vi "Main.Write Data to VS.vi"(8 "error in":errorcluster, 11 "Data Sessions":T1[](array[typedef]) {"Trigger.Refs"."Data Reference" format="%.0x"; "Disable.Refs"."Data Reference" format="%.0x"; "Timing.Refs"."Data Reference" format="%.0x"; "Network"."Name" format="%.0x"; "Incoming.Refs"."Data Reference" format="%.0x"; "Outgoing.Refs"."Data Reference" format="%.0x"}) -> (0 "error out":errorcluster, 3 "Data Sessions out":T1[](array[typedef]) {"Trigger.Refs"."Data Reference" format="%.0x"; "Disable.Refs"."Data Reference" format="%.0x"; "Timing.Refs"."Data Reference" format="%.0x"; "Network"."Name" format="%.0x"; "Incoming.Refs"."Data Reference" format="%.0x"; "Outgoing.Refs"."Data Reference" format="%.0x"})   [LabVIEW 2015, in "J1939 Addon Engine.lvlib"]
uses:
  J1939 Addon Engine.lvlib
  Types/Protocol.XNET Refs.ctl
  Shared/Types/Monitor Settings.ctl
  <vilib>/NI Veristand/Custom Device API/Block Data Reference.ctl
  <vilib>/NI Veristand/Custom Device API/Data Reference.ctl
  Types/Main.Outgoing.Frame.Settings.ctl
  Shared/Types/Outgoing Event Trigger Types.ctl
  <vilib>/NI Veristand/Custom Device API/Global Data Refs.vi
  <vilib>/xnet/xnet.llb/XNET Read (Signal XY).vi
  <vilib>/xnet/xnet.llb/XNET Read (Signal Single-point).vi
  <vilib>/NI Veristand/Custom Device API/Custom Device API.lvlib
  Shared/J1939 Addon Shared.lvlib
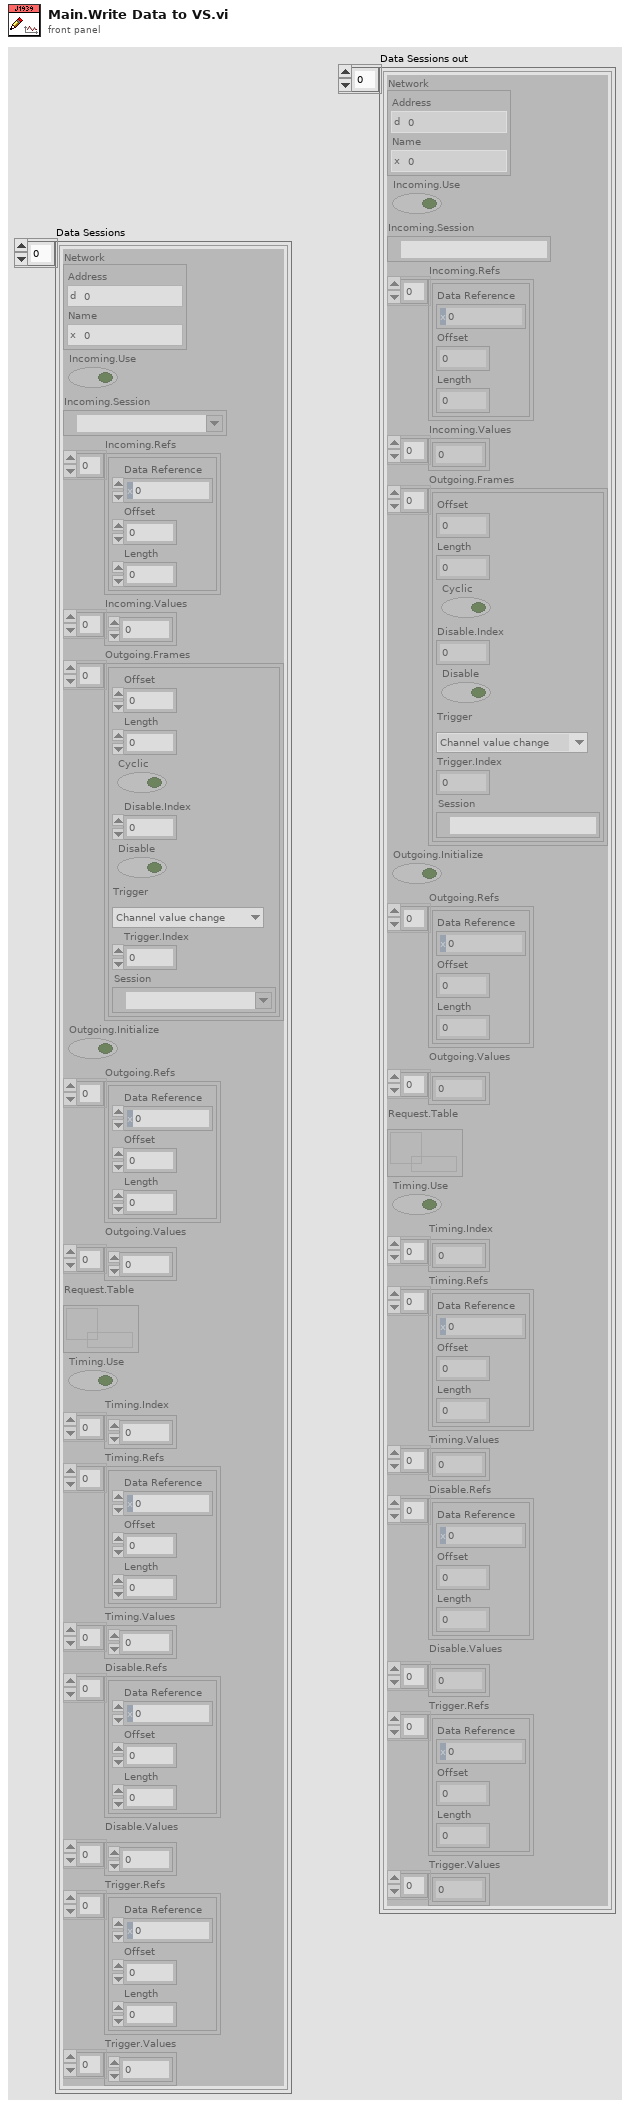
[diagram p1: front panel]
types:
  T1 = typedef "J1939 Addon Engine.lvlib/Protocol.XNET Refs.ctl" = cluster{"Network":T2, "Incoming.Use":bool, "Incoming.Session":refnum<k21>, "Incoming.Refs":T3[], "Incoming.Values":dbl[], "Outgoing.Frames":T5[], "Outgoing.Initialize":bool, "Outgoing.Refs":T3[], "Outgoing.Values":dbl[], "Request.Table":refnum<k33>, "Timing.Use":bool, "Timing.Index":i32[], "Timing.Refs":T3[], "Timing.Values":dbl[], "Disable.Refs":T3[], "Disable.Values":dbl[], "Trigger.Refs":T3[], "Trigger.Values":dbl[]}
  T2 = typedef "J1939 Addon Shared.lvlib/Monitor Settings.ctl" = cluster{"Address":u8, "Name":u64}
  T3 = typedef "Custom Device API.lvlib/Block Data Reference.ctl" = cluster{"Data Reference":T4, "Offset":u64, "Length":u64}
  T4 = typedef "Custom Device API.lvlib/Data Reference.ctl" = i32
  T5 = typedef "J1939 Addon Engine.lvlib/Main.Outgoing.Frame.Settings.ctl" = cluster{"Offset":u32, "Length":u32, "Cyclic":bool, "Disable.Index":i32, "Disable":bool, "Trigger":T6, "Trigger.Index":i32, "Session":refnum<k21>}
  T6 = typedef "J1939 Addon Shared.lvlib/Outgoing Event Trigger Types.ctl" = enum16{"Channel value change", "Trigger channel (not zero)", "Channel value change or trigger channel (not zero)", "Trigger channel (any value change)", "Channel value change or trigger channel (any value change)"}
  T7 = cluster{"timestamp":timestamp[], "value":dbl[]}[]
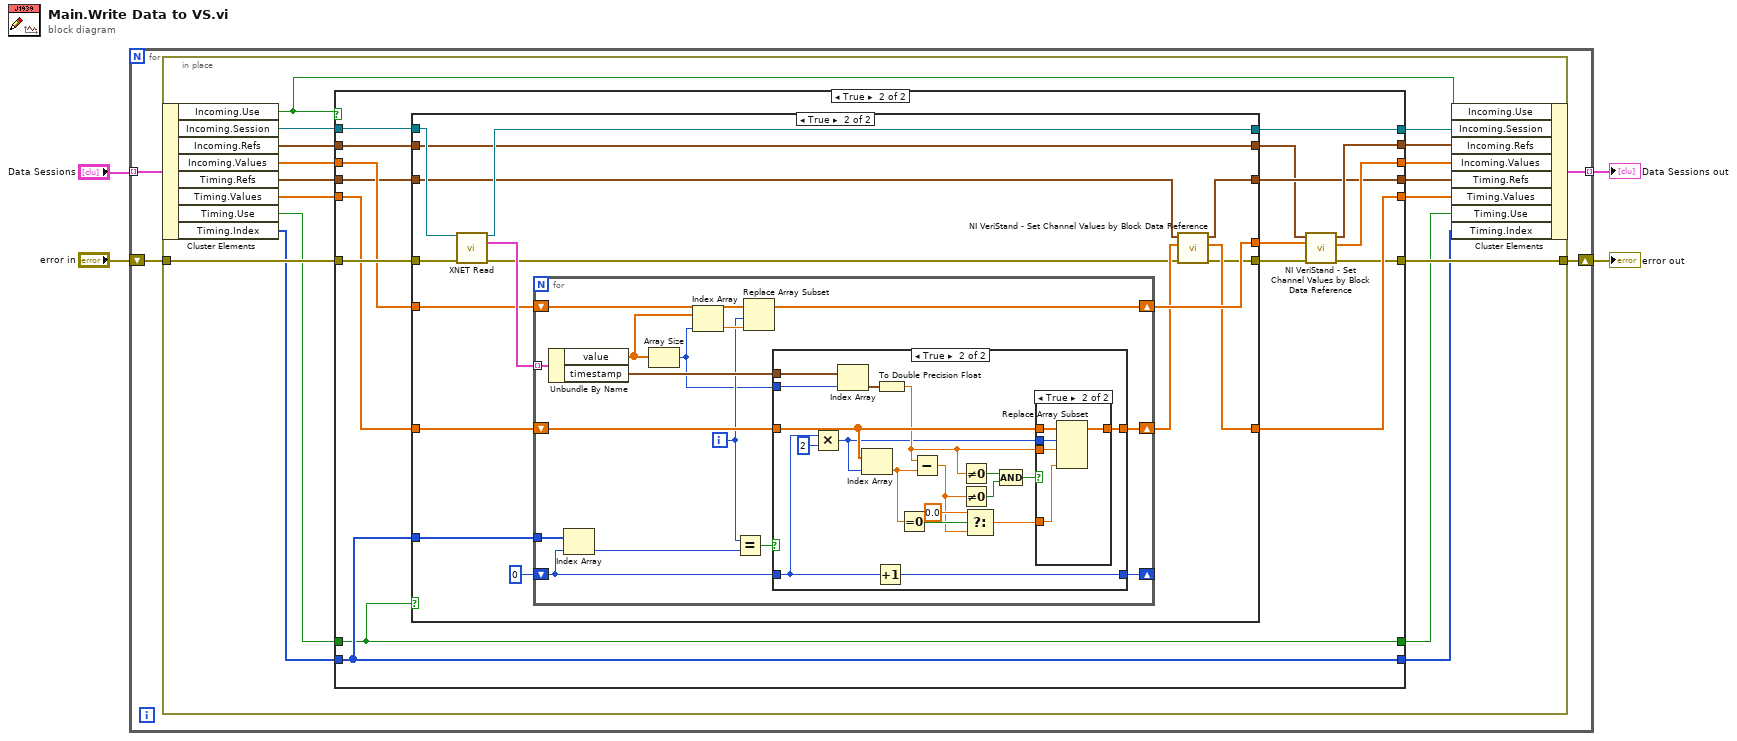
[diagram p0: block diagram]
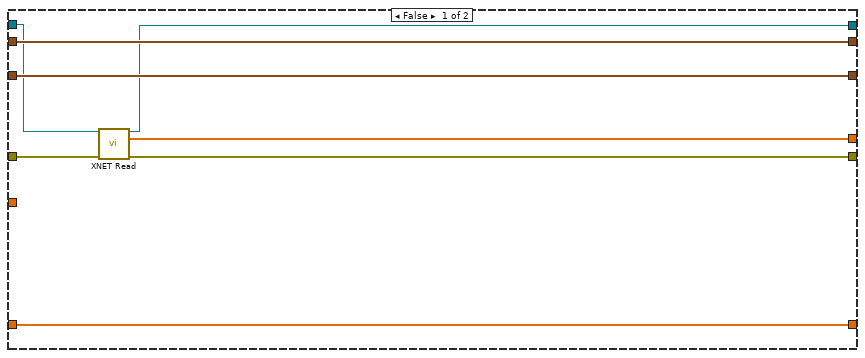
[diagram p3: hidden frame]
diagram:
  n1 = for {
    shift-right: [w7] -> w4
    shift-left: "error in" -> [w8]
    tunnel: "Data Sessions" -> [w6] mode=indexing
    tunnel: [w5] -> w1 mode=indexing
    n2 = in-place {
      in-place-border: w8 -> [w25]
      in-place-border: [w24] -> w7
      n3 = in-place-cluster #1(w6) -> ("Incoming.Use"=w17:bool, "Incoming.Session"=w22:refnum<k21>, "Incoming.Refs"=w21:T3[], "Incoming.Values"=w18:dbl[], "Timing.Refs"=w14:T3[], "Timing.Values"=w16:dbl[], "Timing.Use"=w10:bool, "Timing.Index"=w12:i32[])
      n4 = case shown="True" w17 {
        tunnel: w25 -> [w32 w50]
        tunnel: [w32 w37] -> w24
        tunnel: [w33 w46] -> w23
        tunnel: w22 -> [w30 w49]
        tunnel: w21 -> [w31 w35]
        tunnel: [w30 w48] -> w20
        tunnel: [w31 w47] -> w19
        tunnel: w18 -> [w33 w45]
        tunnel: w16 -> [w29 w43]
        tunnel: [w29 w42] -> w15
        tunnel: w14 -> [w28 w41]
        tunnel: [w28 w40] -> w13
        tunnel: w12 -> [w27 w39]
        tunnel: [w27 w39] -> w11
        tunnel: w10 -> [w26 w34]
        tunnel: [w26 w34] -> w9
        frame False {
        }
        frame True {
          n5 = case shown="True" w34 {
            tunnel: w50 -> [w56 w74]
            tunnel: w49 -> [w55 w73]
            tunnel: [w52 w72] -> w48
            tunnel: w45 -> [_ w70]
            tunnel: [w54 w69] -> w44
            tunnel: w43 -> [w51 w68]
            tunnel: [w51 w66] -> w42
            tunnel: w41 -> [w57 w65]
            tunnel: [w57 w64] -> w40
            tunnel: w39 -> [_ w62]
            tunnel: [w53 w60] -> w38
            tunnel: [w58 w59] -> w36
            tunnel: w35 -> [w58 w59]
            frame False {
              n6 = call-poly <vilib>:"XNET Read.vi"("session in"=w55, "error in (no error)"=w56) -> ("session out"=w52:refnum<k21>, "data"=w54:dbl[], "error out"=w53:errorcluster)  [unwired: 11 in]
            }
            frame True {
              n7 = call-poly <vilib>:"XNET Read.vi"("session in"=w73, "error in (no error)"=w74) -> ("session out"=w72:refnum<k21>, "data"=w71:T7, "error out"=w61:errorcluster)  [unwired: 11 in]
              n8 = for {
                tunnel: w71 -> [w89] mode=indexing
                shift-right: [w87] -> w69
                shift-left: w70 -> [w88]
                shift-right: [w83] -> w67
                shift-left: w68 -> [w84]
                shift-right: [w78] -> _
                shift-left: 0 -> [w81]
                tunnel: w62 -> [w79]
                i -> [w82]
                n9 = Unbundle By Name(w89) -> ("value"=w76:dbl[], "timestamp"=w85:timestamp[])
                n10 = Index Array(array=w79, index=w81) -> (element=w80:i32)
                n11 = Array Size(array=w76) -> (size(s)=w75:i32)
                n12 = Index Array(array=w76, index=w75) -> (element=w86:dbl)
                n13 = Equal?(x=w82, y=w80) -> (x = y?=w77:bool)
                n14 = Replace Array Subset(array=w88, new element=w86, index=w82) -> (w87:dbl[])
                n15 = case shown="True" w77 {
                  tunnel: w85 -> [_ w109]
                  tunnel: w84 -> [w90 w107]
                  tunnel: [w90 w106] -> w83
                  tunnel: w81 -> [w91 w100]
                  tunnel: [w91 w101] -> w78
                  tunnel: w75 -> [_ w92]
                  frame False {
                  }
                  frame True {
                    n16 = Multiply(x=w100, y=2) -> (x*y=w98:i32)
                    n17 = Index Array(array=w109, index=w92) -> (element=w108:timestamp)
                    n18 = Index Array(array=w107, index=w98) -> (element=w97:dbl)
                    n19 = Increment(x=w100) -> (x+1=w101:i32)
                    n20 = To Double Precision Float(number=w108) -> (double precision float=w105:dbl)
                    n21 = Equal To 0?(x=w97) -> (x = 0?=w96:bool)
                    n22 = Subtract(x=w105, y=w97) -> (x-y=w93:dbl)
                    n23 = Not Equal To 0?(x=w105) -> (x != 0?=w104:bool)
                    n24 = Not Equal To 0?(x=w93) -> (x != 0?=w103:bool)
                    n25 = Select(t=0.0, s=w96, f=w93) -> (s? t:f=w94:dbl)
                    n26 = Compound Arithmetic op=AND(w104, w103) -> (w102:bool)
                    n27 = case shown="True" w102 {
                      tunnel: w107 -> [w110 w115]
                      tunnel: w98 -> [_ w114]
                      tunnel: [w110 w113] -> w106
                      tunnel: w94 -> [_ w112]
                      tunnel: w105 -> [_ w111]
                      frame False {
                      }
                      frame True {
                        n28 = Replace Array Subset(array=w115, new element #1=w111, index #1=w114, new element #2=w112) -> (w113:dbl[])  [unwired: 1 in]
                      }
                    }
                  }
                }
              }
              n29 = call <vilib>:"NI VeriStand - Set Channel Values by Block Data Reference.vi"("error in (no error)"=w61, "Values Array in"=w67, "Block Data Ref"=w65) -> ("error out"=w60:errorcluster, "Values Array out"=w66:dbl[], "Block Data Ref dup"=w64:T3[])  [unwired: 6 in]
            }
          }
          n30 = call <vilib>:"NI VeriStand - Set Channel Values by Block Data Reference.vi"("error in (no error)"=w38, "Values Array in"=w44, "Block Data Ref"=w36) -> ("error out"=w37:errorcluster, "Values Array out"=w46:dbl[], "Block Data Ref dup"=w47:T3[])  [unwired: 6 in]
        }
      }
      n31 = in-place-cluster #1("Incoming.Use"=w17, "Incoming.Session"=w20, "Incoming.Refs"=w19, "Incoming.Values"=w23, "Timing.Refs"=w13, "Timing.Values"=w15, "Timing.Use"=w9, "Timing.Index"=w11) -> (w5:T1)
    }
  }
  "error out" <- w4
  "Data Sessions out" <- w1
